vi "Read Physical Address.vi"(11 "Toggle 6 in":refnum<class "Toggle 6.lvclass">) -> (2 "Physical Adress":u32, 3 "Toggle 6 out":refnum<class "Toggle 6.lvclass">)   [LabVIEW 2020, in "Toggle 6.lvclass"]
uses:
  Toggle 6.lvclass
  Toggle 6.lvclass/Toggle 6.ctl
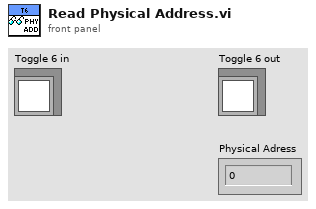
[diagram p1: front panel]
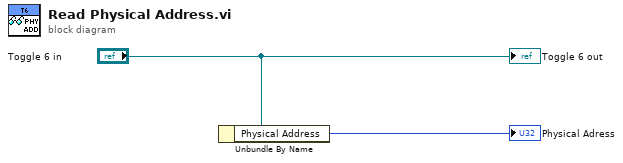
[diagram p0: block diagram]
diagram:
  n1 = Unbundle By Name("Toggle 6 in") -> ("Physical Address"=→"Physical Adress":u32)
  "Toggle 6 out" <- "Toggle 6 in"
